vi "editTreeElement(Req).vi"(8 "error in (no error)":errorcluster, 9 "Req":string, 10 "Active Item:Tag":string, 11 "Tree Control in":refnum<vi>) -> (0 "error out":errorcluster)   [LabVIEW 2010]
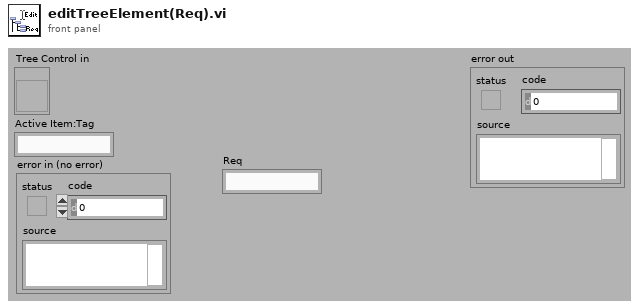
[diagram p1: front panel]
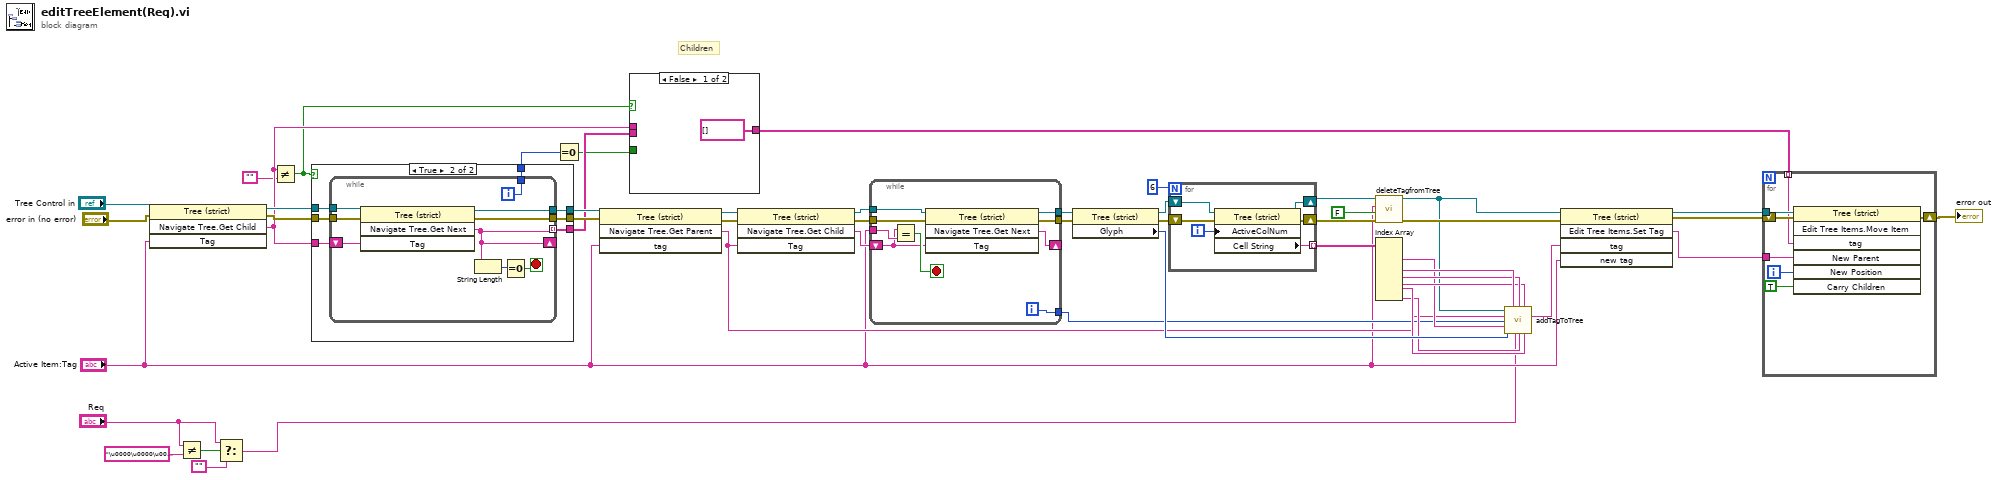
[diagram p0: block diagram]
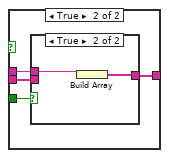
[diagram p2: hidden frame]
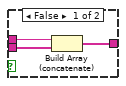
[diagram p3: hidden frame]
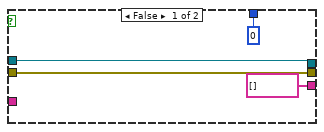
[diagram p4: hidden frame]
diagram:
  # "Children"
  n1 = invoke class="Tree (strict)" method="Navigate Tree.Get Child"(reference="Tree Control in", error in="error in (no error)", "Tag"="Active Item:Tag") -> (reference out=w20:refnum<vi>, error out=w19:errorcluster, "Navigate Tree:Get Child"=w8:string)  [unwired: 1 in, 1 out]
  n2 = Not Equal?(x="Req", y="\u0000\u0000\u0000\u0000") -> (x != y?=w4:bool)
  n3 = Select(t="Req", s=w4, f="") -> (s? t:f=w3:string)
  n4 = Not Equal?(x=w8, y="") -> (x != y?=w6:bool)
  n5 = case shown="True" w6 {
    tunnel: w20 -> [w53 w60]
    tunnel: w19 -> [w52 w59]
    tunnel: [w53 w58] -> w18
    tunnel: [w52 w57] -> w17
    tunnel: [string[] [] w56] -> w16
    tunnel: [0 w55] -> w9
    tunnel: w8 -> [_ w54]
    frame False {
    }
    frame True {
      n6 = while {
        tunnel: w60 -> [w69]
        shift-right: [w62] -> _
        shift-left: w54 -> [w68]
        tunnel: w59 -> [w67]
        tunnel: [w66] -> w57
        tunnel: [w65] -> w58
        tunnel: [w62] -> w56 mode=indexing
        tunnel: [w61] -> w55
        i -> [w61]
        stop <- w63 stop-if-true
        n7 = invoke class="Tree (strict)" method="Navigate Tree.Get Next"(reference=w69, error in=w67, "Tag"=w68) -> (reference out=w65:refnum<vi>, error out=w66:errorcluster, "Navigate Tree:Get Next Item"=w62:string)  [unwired: 1 in, 1 out]
        n8 = String Length(string=w62) -> (length=w64:i32)
        n9 = Equal To 0?(x=w64) -> (x = 0?=w63:bool)
      }
    }
  }
  n10 = Equal To 0?(x=w9) -> (x = 0?=w10:bool)
  n11 = invoke class="Tree (strict)" method="Navigate Tree.Get Parent"(reference=w18, error in=w17, "tag"="Active Item:Tag") -> (reference out=w26:refnum<vi>, error out=w28:errorcluster, "Navigate Tree:Get Parent"=w30:string)  [unwired: 1 in, 1 out]
  n12 = case shown="False" w6 {
    tunnel: w16 -> [_ w74]
    tunnel: [string[] [] w73] -> w11
    tunnel: w10 -> [_ w72]
    tunnel: w8 -> [_ w71]
    frame False {
    }
    frame True {
      n13 = case shown="True" w72 {
        tunnel: w71 -> [w77 w79]
        tunnel: w74 -> [w76 _]
        tunnel: [w75 w78] -> w73
        frame False {
          n14 = Build Array (concatenate)(w77, w76) -> (w75:string[])
        }
        frame True {
          n15 = Build Array(w79) -> (w78:string[])
        }
      }
    }
  }
  n16 = invoke class="Tree (strict)" method="Navigate Tree.Get Child"(reference=w26, error in=w28, "Tag"=w30) -> (reference out=w31:refnum<vi>, error out=w29:errorcluster, "Navigate Tree:Get Child"=w32:string)  [unwired: 1 in, 1 out]
  n17 = while {
    tunnel: "Active Item:Tag" -> [w88]
    tunnel: [w86] -> w33
    tunnel: w31 -> [w85]
    shift-right: [w84] -> _
    shift-left: w32 -> [w83]
    tunnel: w29 -> [w82]
    tunnel: [w81] -> w27
    tunnel: [w80] -> w25
    i -> [w86]
    stop <- w87 stop-if-true
    n18 = Equal?(x=w83, y=w88) -> (x = y?=w87:bool)
    n19 = invoke class="Tree (strict)" method="Navigate Tree.Get Next"(reference=w85, error in=w82, "Tag"=w83) -> (reference out=w80:refnum<vi>, error out=w81:errorcluster, "Navigate Tree:Get Next Item"=w84:string)  [unwired: 1 in, 1 out]
  }
  n20 = property class="Tree (strict)"(reference=w25, error in=w27) -> (reference out=w47:refnum<vi>, error out=w46:errorcluster, "Glyph"=w48:i32)
  n21 = for {
    N: 6 -> [_]
    tunnel: [w91] -> w44 mode=indexing
    shift-right: [w89] -> w24
    shift-left: w47 -> [w94]
    shift-right: [w90] -> w37
    shift-left: w46 -> [w93]
    i -> [w92]
    n22 = property class="Tree (strict)"(reference=w94, error in=w93, "ActiveColNum"=w92) -> (reference out=w89:refnum<vi>, error out=w90:errorcluster, "Cell String"=w91:string)
  }
  n23 = call "deleteTagfromTree.vi"("error in (no error)"=w37, "Delete Children?"=FALSE, "Tag"="Active Item:Tag", "Tree Ref"=w24) -> ("error out"=w38:errorcluster, "Tree ref out"=w36:refnum<vi>)  [unwired: 6 in]
  n24 = Index Array(array=w44) -> (element #1=w34:string, element #3=w43:string, element #4=w42:string, element #5=w41:string, element #6=w40:string, element #7=w39:string)  [unwired: 7 in, 1 out]
  n25 = call "addTagToTree.vi"("Tree ref"=w36, "Element name"=w43, "Calibration path"=w42, "Stimulus path"=w41, "parent tag"=w30, "Child Position"=w33, "new tag"=w34, "Symbol"=w48, "Req"=w3, "Req doc path"=w39, "Analysis script path"=w40) -> ("New Element Tag"=w35:string)  [unwired: 4 in]
  n26 = invoke class="Tree (strict)" method="Edit Tree Items.Set Tag"(reference=w36, error in=w38, "tag"=w35, "new tag"="Active Item:Tag") -> (reference out=w13:refnum<vi>, error out=w14:errorcluster, "Edit Tree Items:Set Tag"=w12:string)  [unwired: 1 in, 2 out]
  n27 = for {
    tunnel: w13 -> [w99]
    tunnel: w12 -> [w98]
    tunnel: w11 -> [w97] mode=indexing
    shift-right: [w101] -> w15
    shift-left: w14 -> [w100]
    i -> [w96]
    n28 = invoke class="Tree (strict)" method="Edit Tree Items.Move Item"(reference=w99, error in=w100, "tag"=w97, "New Parent"=w98, "New Position"=w96, "Carry Children"=TRUE ("Carry Children?")) -> (error out=w101:errorcluster)  [unwired: 1 in, 6 out]
  }
  "error out" <- w15
